vi "Angle_Calibration_fit.vi"(0 "Reference Velocity":dbl[](array[numeric])=[14.0, 14.0, 14.0, 14.0, 14.0, 14.0, 14.0, 14.0, 14.0, 14.0, 14.0, 14.0] format="%.2f", 4 "Vel calib file":path=path "C:/Documents and Settings/Paul Nathan/Desktop/XW207_14ms_190708.xls", 5 "coeff suffix":string="1", 6 "Point selector":cluster{"Y":dbl, "X":dbl, "switch":bool}[](array[cluster])=[{"Y"=4.15, "X"=-20.0, "switch"=FALSE}, {"Y"=4.14, "X"=-20.0, "switch"=TRUE}, {"Y"=5.05, "X"=-15.0, "switch"=FALSE}, {"Y"=5.89, "X"=-10.0, "switch"=FALSE}, {"Y"=6.62, "X"=-5.0, "switch"=FALSE}, {"Y"=7.22, "X"=0.0, "switch"=FALSE}, {"Y"=7.22, "X"=0.0, "switch"=FALSE}, {"Y"=7.78, "X"=5.0, "switch"=FALSE}, {"Y"=8.23, "X"=10.0, "switch"=FALSE}, {"Y"=8.6, "X"=15.0, "switch"=FALSE}, {"Y"=8.9, "X"=20.0, "switch"=FALSE}, {"Y"=4.14, "X"=20.0, "switch"=TRUE}] {"X" format="%.2f"; "Y" format="%.3f"}, 7 "Angle":dbl[](array[numeric])=[-20.0, -20.0, -15.0, -10.0, -5.0, 0.0, 0.0, 5.0, 10.0, 15.0, 20.0, 20.0] format="%.2f", 8 "HW voltage":dbl[](array[numeric])=[4.15, 4.14, 5.05, 5.89, 6.62, 7.22, 7.22, 7.78, 8.23, 8.6, 8.9, 4.14] format="%.4f") -> (1 "Calib const":string[][](array[string])=[["psi1"], ["43.668881224145"]], 2 "Angle calibration (output)":cluster{cluster{"Y":dbl, "Y":dbl}[]}[](graph)=[{[{"Y"=-0.3707430055212287, "Y"=0.35390163729735447}, {"Y"=-0.27435540227684596, "Y"=0.26189254960381586}, {"Y"=-0.18248651716481784, "Y"=0.17419691217678165}, {"Y"=-0.09350499943039396, "Y"=0.0892574802088237}, {"Y"=-0.005967517864122852, "Y"=0.005696487437982681}, {"Y"=-0.005967517864122852, "Y"=0.005696487437982681}, {"Y"=0.08147860648290228, "Y"=-0.07777729811829852}, {"Y"=0.17018039317919034, "Y"=-0.16244970614591436}, {"Y"=0.2615634368305997, "Y"=-0.24968157200844676}, {"Y"=0.35722682015059526, "Y"=-0.3409993382841948}]}, {[{"Y"=-0.3707430055212287, "Y"=0.3491582385529654}, {"Y"=-0.27435540227684596, "Y"=0.2651280690077785}, {"Y"=-0.18248651716481784, "Y"=0.17628323511940247}, {"Y"=-0.09350499943039396, "Y"=0.08922339098301249}, {"Y"=-0.005967517864122852, "Y"=0.00788326539441427}, {"Y"=-0.005967517864122852, "Y"=0.00788326539441427}, {"Y"=0.08147860648290228, "Y"=-0.08034320825038008}, {"Y"=0.17018039317919034, "Y"=-0.16502077054753508}, {"Y"=0.2615634368305997, "Y"=-0.2507383378676811}, {"Y"=0.35722682015059526, "Y"=-0.3397235081805045}]}], 3 "Point selector":cluster{"Y":dbl, "X":dbl, "switch":bool}[](array[cluster])=[{"Y"=4.15, "X"=-20.0, "switch"=FALSE}, {"Y"=4.14, "X"=-20.0, "switch"=TRUE}, {"Y"=5.05, "X"=-15.0, "switch"=FALSE}, {"Y"=5.89, "X"=-10.0, "switch"=FALSE}, {"Y"=6.62, "X"=-5.0, "switch"=FALSE}, {"Y"=7.22, "X"=0.0, "switch"=FALSE}, {"Y"=7.22, "X"=0.0, "switch"=FALSE}, {"Y"=7.78, "X"=5.0, "switch"=FALSE}, {"Y"=8.23, "X"=10.0, "switch"=FALSE}, {"Y"=8.6, "X"=15.0, "switch"=FALSE}, {"Y"=8.9, "X"=20.0, "switch"=FALSE}, {"Y"=4.14, "X"=20.0, "switch"=TRUE}] {"X" format="%.2f"; "Y" format="%.2f"})   [LabVIEW 2010]
uses:
  Globals/Calib_global.vi
  <vilib>/Analysis/NI_AALPro.lvlib
panel:
  out "Angle calibration":cluster{cluster{"Y":dbl, "Y":dbl}[]}[](graph)=[{[{"Y"=-0.36397023426620234, "Y"=0.3553194647823972}, {"Y"=-0.2679491924311227, "Y"=0.2630881239782155}, {"Y"=-0.17632698070846498, "Y"=0.1750820028913465}, {"Y"=-0.08748866352592401, "Y"=0.089749903260456}, {"Y"=0.0, "Y"=0.005714189963144827}, {"Y"=0.0, "Y"=0.005714189963144827}, {"Y"=0.08748866352592401, "Y"=-0.07832152333416635}, {"Y"=0.17632698070846498, "Y"=-0.16365362296505687}, {"Y"=0.2679491924311227, "Y"=-0.25165974405192587}, {"Y"=0.36397023426620234, "Y"=-0.34389108485610753}]}, {[{"Y"=-0.36397023426620234, "Y"=0.35058342929792774}, {"Y"=-0.2679491924311227, "Y"=0.26631618663669254}, {"Y"=-0.17632698070846498, "Y"=0.1771646292169042}, {"Y"=-0.08748866352592401, "Y"=0.08971510654683099}, {"Y"=0.0, "Y"=0.007900930190801528}, {"Y"=0.0, "Y"=0.007900930190801528}, {"Y"=0.08748866352592401, "Y"=-0.08088799908597503}, {"Y"=0.17632698070846498, "Y"=-0.16622588028036078}, {"Y"=0.2679491924311227, "Y"=-0.25271595275026465}, {"Y"=0.36397023426620234, "Y"=-0.3426094803319098}]}, {[{"Y"=-0.3707430055212287, "Y"=0.35390163729735447}, {"Y"=-0.27435540227684596, "Y"=0.26189254960381586}, {"Y"=-0.18248651716481784, "Y"=0.17419691217678165}, {"Y"=-0.09350499943039396, "Y"=0.0892574802088237}, {"Y"=-0.005967517864122852, "Y"=0.005696487437982681}, {"Y"=-0.005967517864122852, "Y"=0.005696487437982681}, {"Y"=0.08147860648290228, "Y"=-0.07777729811829852}, {"Y"=0.17018039317919034, "Y"=-0.16244970614591436}, {"Y"=0.2615634368305997, "Y"=-0.24968157200844676}, {"Y"=0.35722682015059526, "Y"=-0.3409993382841948}]}, {[{"Y"=-0.3707430055212287, "Y"=0.3491582385529654}, {"Y"=-0.27435540227684596, "Y"=0.2651280690077785}, {"Y"=-0.18248651716481784, "Y"=0.17628323511940247}, {"Y"=-0.09350499943039396, "Y"=0.08922339098301249}, {"Y"=-0.005967517864122852, "Y"=0.00788326539441427}, {"Y"=-0.005967517864122852, "Y"=0.00788326539441427}, {"Y"=0.08147860648290228, "Y"=-0.08034320825038008}, {"Y"=0.17018039317919034, "Y"=-0.16502077054753508}, {"Y"=0.2615634368305997, "Y"=-0.2507383378676811}, {"Y"=0.35722682015059526, "Y"=-0.3397235081805045}]}]
  out "...and this should be very close to psi":dbl=43.66863209489197
  out "If correction worked, this should be tiny...":dbl=5.080099392876688e-08 format="%#_4e"
  out "un-corrected psi (deg)":dbl=43.84673677322887
  out "systematic yaw angle error (deg)":dbl=-0.3419095292109124
  in  "switch":cluster{"Y":dbl, "X":dbl, "switch":bool} {"X" format="%.2f"; "Y" format="%.2f"}
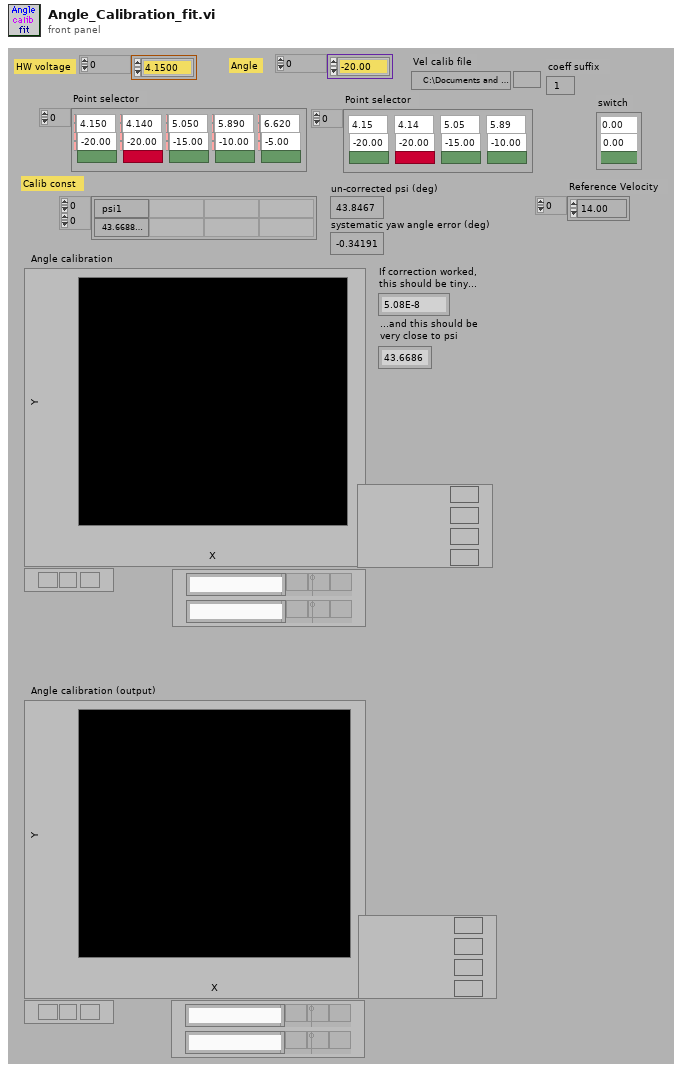
[diagram p1: front panel]
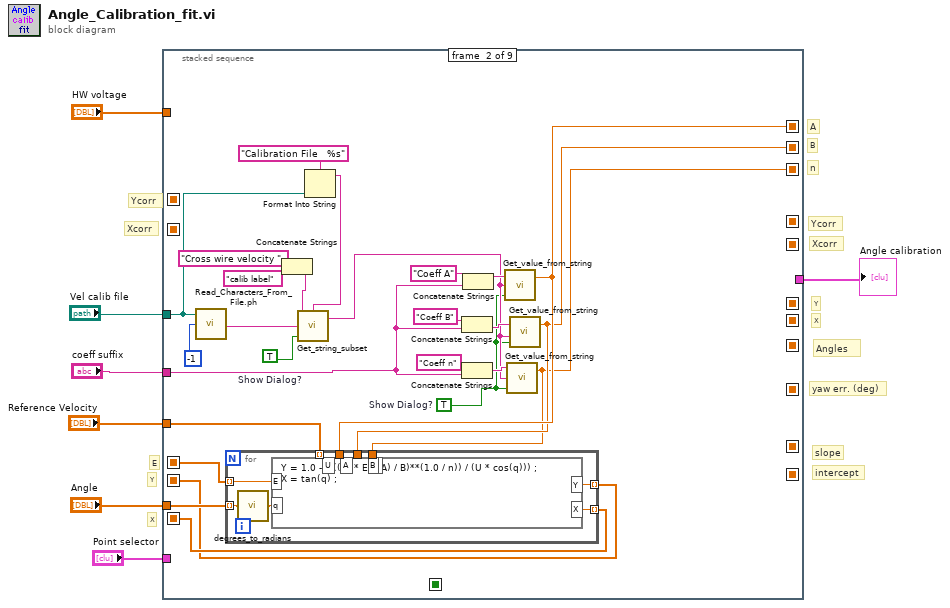
[diagram p0: block diagram]
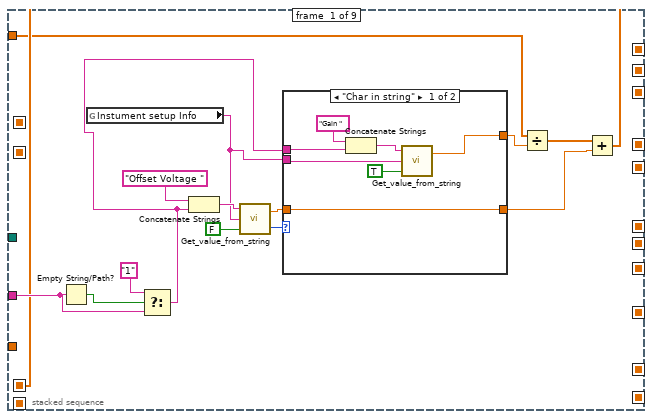
[diagram p2: hidden frame]
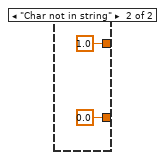
[diagram p3: hidden frame]
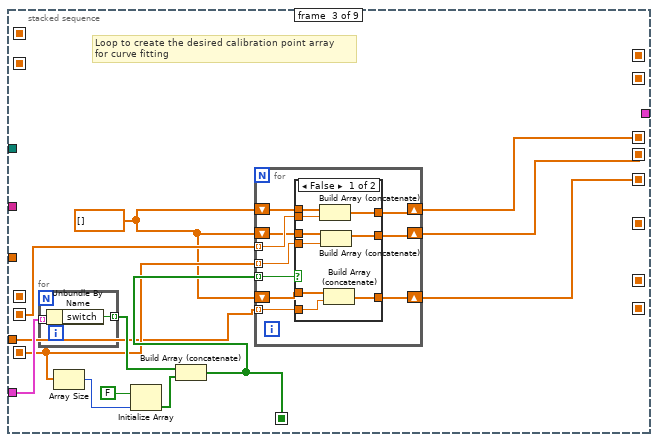
[diagram p4: hidden frame]
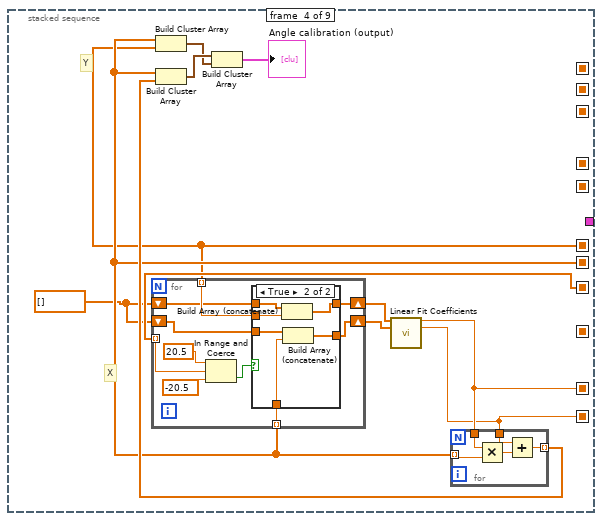
[diagram p6: hidden frame]
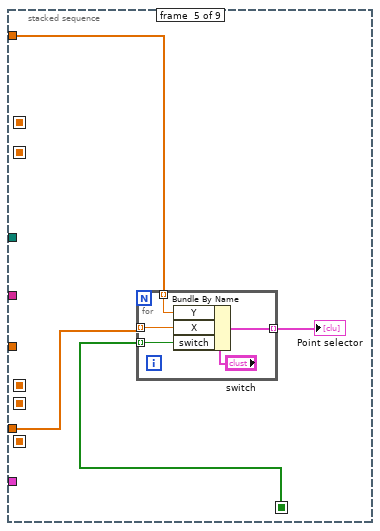
[diagram p8: hidden frame]
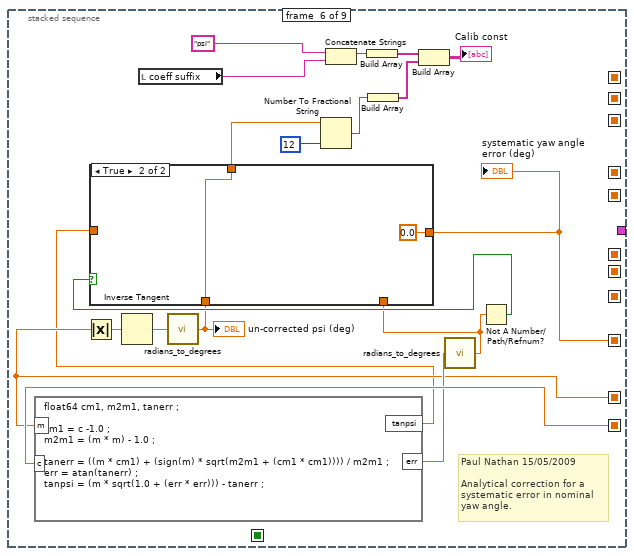
[diagram p9: hidden frame]
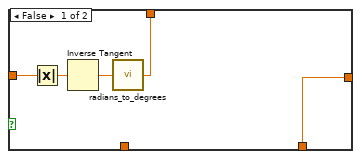
[diagram p10: hidden frame]
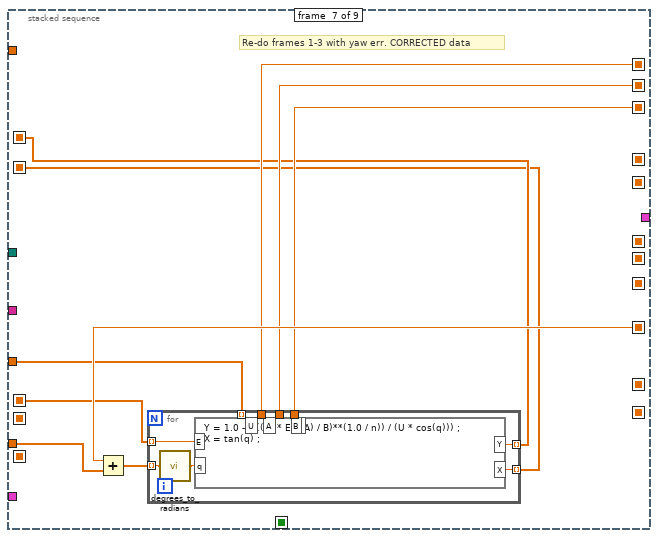
[diagram p11: hidden frame]
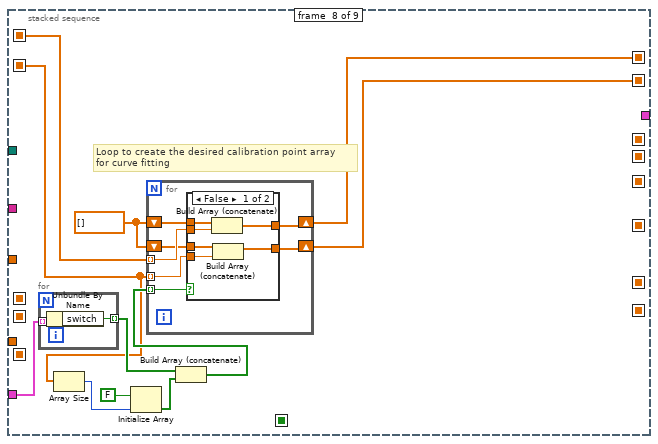
[diagram p12: hidden frame]
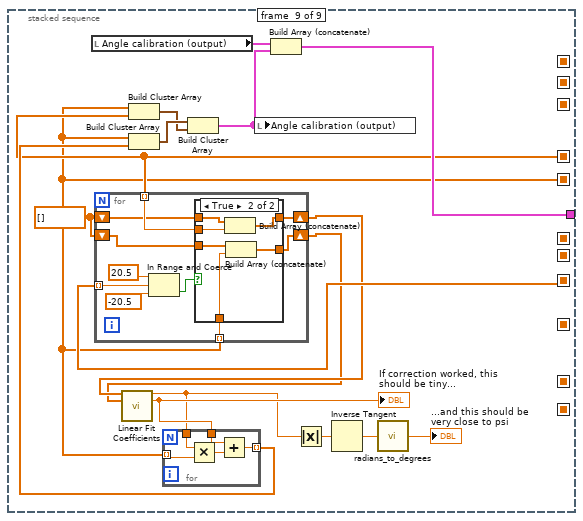
[diagram p14: hidden frame]
diagram:
  # "Angles"
  # "Xcorr"
  # "Ycorr"
  # "yaw err. (deg)"
  # "Xcorr"
  # "Ycorr"
  # "n"
  # "B"
  # "A"
  # "intercept"
  # "E"
  # "slope"
  # "X"
  # "Y"
  # "X"
  # "Y"
  n1 = stacked-sequence "E^2" {
    seq-local: [_ _ _ w115 _ _ _ _ _] -> [_ _ _ _ _ w155 _ _ _]
    seq-local: [_ _ w79 _ _ _ _ _ _] -> [_ _ _ w107 _ _ _ _ _]
    seq-local: [_ _ w78 _ _ _ _ _ _] -> [_ _ _ w108 _ _ _ _ _]
    seq-local: [_ _ w74 _ _ _ _ _ _] -> [_ _ _ _ w141 _ _ _ _]
    seq-local: [_ w46 _ _ _ _ _ _ _] -> [_ _ w71 _ _ _ _ _ _]
    seq-local: [_ w48 _ _ _ _ _ _ _] -> [_ _ w70 _ _ _ _ _ _]
    seq-local: [w9 _ _ _ _ _ _ _ _] -> [_ w39 _ _ _ _ w180 _ _]
    seq-local: [_ _ _ w114 _ _ _ _ _] -> [_ _ _ _ _ w159 _ _ _]
    seq-local: [_ w38 _ _ _ _ _ _ _] -> [_ _ _ _ _ _ w178 _ _]
    seq-local: [_ w37 _ _ _ _ _ _ _] -> [_ _ _ _ _ _ w177 _ _]
    seq-local: [_ w36 _ _ _ _ _ _ _] -> [_ _ _ _ _ _ w176 _ _]
    seq-local: [_ _ _ _ _ _ _ w194 _] -> [_ _ _ _ _ _ _ _ w225]
    seq-local: [_ _ _ _ _ _ _ w193 _] -> [_ _ _ _ _ _ _ _ w224]
    seq-local: [_ _ _ _ _ w149 _ _ _] -> [_ _ _ _ _ _ w181 _ _]
    seq-local: [_ _ _ _ _ _ w175 _ _] -> [_ _ _ _ _ _ _ w196 _]
    seq-local: [_ _ _ _ _ _ w174 _ _] -> [_ _ _ _ _ _ _ w195 _]
    seq-local: [_ _ w69 _ _ _ _ _ _] -> [_ _ _ w109 _ _ _ _ w226]
    tunnel: "Angle" -> [_ w47 w68 _ w140 _ w183 _ _]
    tunnel: "Point selector" -> [_ _ w77 _ _ _ _ w203 _]
    tunnel: "Vel calib file" -> [_ w32 _ _ _ _ _ _ _]
    tunnel: "coeff suffix" -> [w20 w40 _ _ _ _ _ _ _]
    tunnel: "HW voltage" -> [w8 _ _ _ w139 _ _ _ _]
    tunnel: "Reference Velocity" -> [_ w35 _ _ _ _ w179 _ _]
    tunnel: [_ _ _ _ _ _ _ _ w227] -> w1
    frame #0 {
      n2 = Empty String/Path?(string/path=w20) -> (empty?=w21:bool)
      n3 = global read "Calib_global.vi" "Instument setup Info"() -> (w17:string)
      n4 = Select(t="1", s=w21, f=w20) -> (s? t:f=w13:string)
      n5 = Concatenate Strings("Offset Voltage ", w13) -> (w19:string)
      n6 = call "Get_value_from_string.vi"("Show Dialog?"=FALSE, "Input string"=w17, "Variable name"=w19) -> ("Status"=w15:enum16{"Char in string", "Char not in string"}, "Value"=w16:dbl)
      n7 = case shown="\"Char in string\"" w15 {
        tunnel: w17 -> [w29 _]
        tunnel: [w27 1.0 ("Value")] -> w11
        tunnel: w16 -> [w26 _]
        tunnel: [w26 0.0 ("Value")] -> w10
        tunnel: w13 -> [w23 _]
        frame "Char in string" {
          n8 = Concatenate Strings("Gain ", w23) -> (w25:string)
          n9 = call "Get_value_from_string.vi"("Show Dialog?"=TRUE, "Input string"=w29, "Variable name"=w25) -> ("Value"=w27:dbl)  [unwired: 1 out]
        }
        frame "Char not in string" {
        }
      }
      n10 = Divide(x=w8, y=w11) -> (x/y=w12:dbl[])
      n11 = Add(x=w12, y=w10) -> (x+y=w9:dbl[])
    }
    frame #1 {
      w41 = TRUE  # Show Dialog?
      w42 = TRUE  # Show Dialog?
      n12 = call "Read_Characters_From_File.ph.vi"("file path (dialog if empty)"=w32, "number of characters (all:-1)"=-1) -> ("character string"=w55:string)  [unwired: 7 out]
      n13 = Concatenate Strings("Cross wire velocity ", "calib label") -> (w57:string)
      n14 = Format Into String(format string="Calibration File   %s", w32) -> (resulting string=w33:string)  [unwired: 2 in, 1 out]
      n15 = call "Get_string_subset.vi"("String Name"=w33, "Show Dialog?"=w41, "String to split"=w55, "File Label"=w57) -> ("Output string"=w43:string)  [unwired: 1 out]
      n16 = Concatenate Strings("Coeff B", w40) -> (w45:string)
      n17 = Concatenate Strings("Coeff n", w40) -> (w49:string)
      n18 = Concatenate Strings("Coeff A", w40) -> (w51:string)
      n19 = call "Get_value_from_string.vi"("Show Dialog?"=w42, "Input string"=w43, "Variable name"=w51) -> ("Value"=w38:dbl)  [unwired: 1 out]
      n20 = call "Get_value_from_string.vi"("Show Dialog?"=w42, "Input string"=w43, "Variable name"=w49) -> ("Value"=w36:dbl)  [unwired: 1 out]
      n21 = call "Get_value_from_string.vi"("Show Dialog?"=w42, "Input string"=w43, "Variable name"=w45) -> ("Value"=w37:dbl)  [unwired: 1 out]
      n22 = for {
        tunnel: w47 -> [w61] mode=indexing
        tunnel: [w66] -> w46 mode=indexing
        tunnel: [w65] -> w48 mode=indexing
        tunnel: w38 -> [w64]
        tunnel: w36 -> [w63]
        tunnel: w37 -> [w60]
        tunnel: w35 -> [w59] mode=indexing
        tunnel: w39 -> [w58] mode=indexing
        n23 = call "degrees_to_radians.vi"("degrees"=w61) -> ("radians"=w62:dbl)
        n24 = formula code="Y = 1.0 - (((((E * E) - A) / B)**(1.0 / n)) / (U * cos(q))) ;\nX = tan(q) ;"("E"=w58, "q"=w62, "A"=w64, "n"=w63, "U"=w59, "B"=w60) -> ("Y"=w66:dbl, "X"=w65:dbl)
      }
    }
    frame #2 {
      w67 = dbl[] []
      # "Loop to create the desired calibration point array\nfor curve fitting"
      n25 = for {
        tunnel: w77 -> [w81] mode=indexing
        tunnel: [w80] -> w76 mode=indexing
        n26 = Unbundle By Name(w81) -> ("switch"=w80:bool)
      }
      n27 = Array Size(array=w70) -> (size(s)=w72:i32)
      n28 = Initialize Array(FALSE, w72) -> (w75:bool[])
      n29 = Build Array (concatenate)(w76, w75) -> (w74:bool[])
      n30 = for {
        shift-right: [w85] -> w78
        shift-left: w67 -> [w87]
        shift-right: [w86] -> w79
        shift-left: w67 -> [w88]
        tunnel: w74 -> [w89] mode=indexing
        tunnel: w70 -> [w90] mode=indexing
        tunnel: w71 -> [w91] mode=indexing
        shift-right: [w83] -> w69
        shift-left: w67 -> [w84]
        tunnel: w68 -> [w82] mode=indexing
        n31 = case shown="False" w89 {
          tunnel: [w95 w102] -> w85
          tunnel: [w96 w103] -> w86
          tunnel: w87 -> [w97 w102]
          tunnel: w88 -> [w98 w103]
          tunnel: w90 -> [w99 _]
          tunnel: w91 -> [w100 _]
          tunnel: w84 -> [w94 w101]
          tunnel: [w93 w101] -> w83
          tunnel: w82 -> [w92 _]
          frame False {
            n32 = Build Array (concatenate)(w98, w100) -> (w96:dbl[])
            n33 = Build Array (concatenate)(w97, w99) -> (w95:dbl[])
            n34 = Build Array (concatenate)(w94, w92) -> (w93:dbl[])
          }
          frame True {
          }
        }
      }
    }
    frame #3 {
      w106 = dbl[] []
      # "X"
      # "Y"
      n35 = for {
        tunnel: w109 -> [w125] mode=indexing
        tunnel: w108 -> [w121] mode=indexing
        tunnel: w107 -> [w120] mode=indexing
        shift-right: [w118] -> w105
        shift-left: w106 -> [w119]
        shift-right: [w117] -> w104
        shift-left: w106 -> [w116]
        n36 = In Range and Coerce(upper limit=20.5, x=w125, lower limit=-20.5) -> (In Range?=w122:bool)  [unwired: 1 out]
        n37 = case shown="True" w122 {
          tunnel: w121 -> [_ w133]
          tunnel: w120 -> [_ w132]
          tunnel: w119 -> [w127 w131]
          tunnel: [w127 w130] -> w118
          tunnel: [w126 w129] -> w117
          tunnel: w116 -> [w126 w128]
          frame False {
          }
          frame True {
            n38 = Build Array (concatenate)(w131, w132) -> (w130:dbl[])
            n39 = Build Array (concatenate)(w128, w133) -> (w129:dbl[])
          }
        }
      }
      n40 = Build Cluster Array(w108, w107) -> (w110:cluster{"Y":dbl, "Y":dbl}[])
      n41 = call <vilib>:"Linear Fit Coefficients.vi"("Y"=w105, "X"=w104) -> ("slope"=w115:dbl, "intercept"=w114:dbl)  [unwired: 3 in, 9 out]
      n42 = for {
        tunnel: w108 -> [w137] mode=indexing
        tunnel: w115 -> [w138]
        tunnel: w114 -> [w135]
        tunnel: [w134] -> w113 mode=indexing
        n43 = Multiply(x=w138, y=w137) -> (x*y=w136:dbl)
        n44 = Add(x=w135, y=w136) -> (x+y=w134:dbl)
      }
      n45 = Build Cluster Array(w108, w113) -> (w111:cluster{"Y":dbl, dbl}[])
      n46 = Build Cluster Array(w111, w110) -> (→"Angle calibration (output)":cluster{cluster{"Y":dbl, "Y":dbl}[]}[])
    }
    frame #4 {
      n47 = for {
        tunnel: w140 -> [w147] mode=indexing
        tunnel: [w146] -> w142 mode=indexing
        tunnel: w141 -> [w145] mode=indexing
        tunnel: w139 -> [w143] mode=indexing
        n48 = Bundle By Name(cluster="switch", "Y"=w143, "X"=w147, "switch"=w145) -> (w146:cluster{"Y":dbl, "X":dbl, "switch":bool})
      }
      "Point selector" <- w142
    }
    frame #5 {
      # "Paul Nathan 15/05/2009\n\nAnalytical correction for a systematic error in nominal yaw angle."
      n49 = formula code="float64 cm1, m2m1, tanerr ;\n\ncm1 = c -1.0 ;\nm2m1 = (m * m) - 1.0 ;\n\ntanerr = ((m * cm1) + (sign(m) * sqrt(m2m1 + (cm1 * cm1)))) / m2m1 ;\nerr = atan(tanerr) ;\ntanpsi = (m * sqrt(1.0 + (err * err))) - tanerr ;"("m"=w155, "c"=w159) -> ("tanpsi"=w152:dbl, "err"=w157:dbl)
      n50 = Absolute Value(x=w155) -> (abs(x)=w156:dbl)
      n51 = Inverse Tangent(1:w156) -> (0:w154:dbl)
      n52 = local read "coeff suffix"() -> (w161:string)
      n53 = call "radians_to_degrees.vi"("radians"=w154) -> ("degrees"=w150:dbl)
      "un-corrected psi (deg)" <- w150
      n54 = Concatenate Strings("psi", w161) -> (w160:string)
      n55 = Build Array(w160) -> (w166:string[])
      n56 = call "radians_to_degrees.vi"("radians"=w157) -> ("degrees"=w148:dbl)
      n57 = Not A Number/Path/Refnum?(number/path/refnum=w148) -> (NaN/Path/Refnum?=w153:bool)
      n58 = case shown="True" w153 {
        tunnel: w152 -> [w169 _]
        tunnel: [w168 w173] -> w151
        tunnel: w150 -> [_ w173]
        tunnel: [w167 0.0 ("degrees")] -> w149
        tunnel: w148 -> [w167 _]
        frame False {
          n59 = Absolute Value(x=w169) -> (abs(x)=w170:dbl)
          n60 = Inverse Tangent(1:w170) -> (0:w171:dbl)
          n61 = call "radians_to_degrees.vi"("radians"=w171) -> ("degrees"=w168:dbl)
        }
        frame True {
        }
      }
      "systematic yaw angle error (deg)" <- w149
      n62 = Number To Fractional String(number=w151, precision (6)=i16 12) -> (F-format string=w164:string)  [unwired: 2 out]
      n63 = Build Array(w164) -> (w163:string[])
      n64 = Build Array(w166, w163) -> (→"Calib const":string[][])
    }
    frame #6 {
      # "Re-do frames 1-3 with yaw err. CORRECTED data"
      n65 = Add(x=w181, y=w183) -> (x+y=w182:dbl[])
      n66 = for {
        tunnel: w182 -> [w189] mode=indexing
        tunnel: [w192] -> w175 mode=indexing
        tunnel: [w191] -> w174 mode=indexing
        tunnel: w177 -> [w188]
        tunnel: w179 -> [w187] mode=indexing
        tunnel: w180 -> [w186] mode=indexing
        tunnel: w178 -> [w185]
        tunnel: w176 -> [w184]
        n67 = call "degrees_to_radians.vi"("degrees"=w189) -> ("radians"=w190:dbl)
        n68 = formula code="Y = 1.0 - (((((E * E) - A) / B)**(1.0 / n)) / (U * cos(q))) ;\nX = tan(q) ;"("E"=w186, "q"=w190, "A"=w185, "n"=w184, "U"=w187, "B"=w188) -> ("Y"=w192:dbl, "X"=w191:dbl)
      }
    }
    frame #7 {
      w197 = dbl[] []
      # "Loop to create the desired calibration point array\nfor curve fitting"
      n69 = for {
        tunnel: w203 -> [w205] mode=indexing
        tunnel: [w204] -> w202 mode=indexing
        n70 = Unbundle By Name(w205) -> ("switch"=w204:bool)
      }
      n71 = Array Size(array=w195) -> (size(s)=w198:i32)
      n72 = Initialize Array(FALSE, w198) -> (w201:bool[])
      n73 = Build Array (concatenate)(w202, w201) -> (w200:bool[])
      n74 = for {
        shift-right: [w206] -> w193
        shift-left: w197 -> [w208]
        shift-right: [w207] -> w194
        shift-left: w197 -> [w209]
        tunnel: w200 -> [w210] mode=indexing
        tunnel: w195 -> [w211] mode=indexing
        tunnel: w196 -> [w212] mode=indexing
        n75 = case shown="False" w210 {
          tunnel: [w213 w219] -> w206
          tunnel: [w214 w220] -> w207
          tunnel: w208 -> [w215 w219]
          tunnel: w209 -> [w216 w220]
          tunnel: w211 -> [w217 _]
          tunnel: w212 -> [w218 _]
          frame False {
            n76 = Build Array (concatenate)(w216, w218) -> (w214:dbl[])
            n77 = Build Array (concatenate)(w215, w217) -> (w213:dbl[])
          }
          frame True {
          }
        }
      }
    }
    frame #8 {
      w223 = dbl[] []
      n78 = local read "Angle calibration (output)"() -> (w229:cluster{cluster{"Y":dbl, "Y":dbl}[]}[])
      n79 = for {
        tunnel: w224 -> [w244] mode=indexing
        tunnel: w225 -> [w243] mode=indexing
        shift-right: [w241] -> w222
        shift-left: w223 -> [w242]
        shift-right: [w240] -> w221
        shift-left: w223 -> [w239]
        tunnel: w226 -> [w238] mode=indexing
        n80 = In Range and Coerce(upper limit=20.5, x=w238, lower limit=-20.5) -> (In Range?=w245:bool)  [unwired: 1 out]
        n81 = case shown="True" w245 {
          tunnel: w244 -> [_ w255]
          tunnel: w243 -> [_ w254]
          tunnel: w242 -> [w249 w253]
          tunnel: [w249 w252] -> w241
          tunnel: [w248 w251] -> w240
          tunnel: w239 -> [w248 w250]
          frame False {
          }
          frame True {
            n82 = Build Array (concatenate)(w253, w254) -> (w252:dbl[])
            n83 = Build Array (concatenate)(w250, w255) -> (w251:dbl[])
          }
        }
      }
      n84 = call <vilib>:"Linear Fit Coefficients.vi"("Y"=w222, "X"=w221) -> ("slope"=w234:dbl, "intercept"=w237:dbl)  [unwired: 3 in, 9 out]
      "If correction worked, this should be tiny..." <- w237
      n85 = Build Cluster Array(w224, w225) -> (w230:cluster{"Y":dbl, "Y":dbl}[])
      n86 = for {
        tunnel: w224 -> [w259] mode=indexing
        tunnel: w234 -> [w260]
        tunnel: w237 -> [w257]
        tunnel: [w256] -> w232 mode=indexing
        n87 = Multiply(x=w260, y=w259) -> (x*y=w258:dbl)
        n88 = Add(x=w257, y=w258) -> (x+y=w256:dbl)
      }
      n89 = Build Cluster Array(w224, w232) -> (w231:cluster{"Y":dbl, dbl}[])
      n90 = Build Cluster Array(w231, w230) -> (w228:cluster{cluster{"Y":dbl, "Y":dbl}[]}[])
      n91 = local write "Angle calibration (output)"(w228) -> ()
      n92 = Build Array (concatenate)(w229, w228) -> (w227:cluster{cluster{"Y":dbl, "Y":dbl}[]}[])
      n93 = Absolute Value(x=w234) -> (abs(x)=w236:dbl)
      n94 = Inverse Tangent(1:w236) -> (0:w235:dbl)
      n95 = call "radians_to_degrees.vi"("radians"=w235) -> ("degrees"=→"...and this should be very close to psi":dbl)
    }
  }
  "Angle calibration" <- w1
